vi "GraphChartFactory.vi"(8 "error in":errorcluster, 11 "Gen Refnum":refnum<vi>) -> (0 "error out":errorcluster, 3 "GraphChart out":refnum<class "GraphChart.lvclass">)   [LabVIEW 2014, in "GraphChart.lvclass"]
uses:
  GraphChart.lvclass
  WaveformChart/WaveformChart.lvclass
  WaveformGraph/WaveformGraph.lvclass
  XYGraph/XYGraph.lvclass
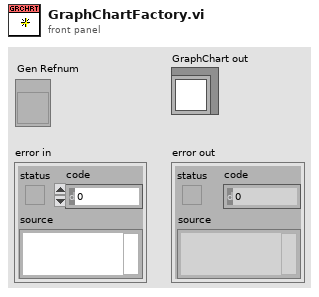
[diagram p1: front panel]
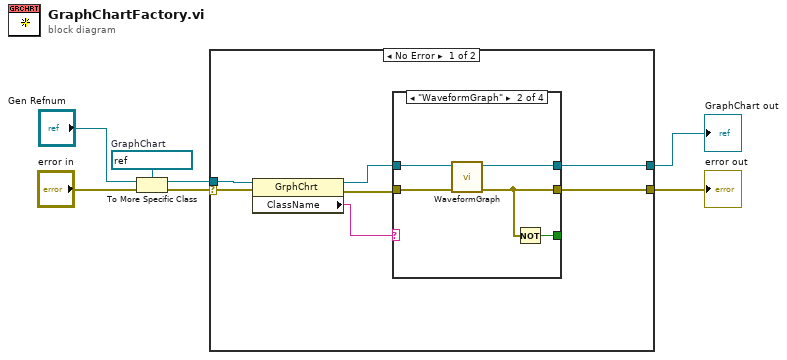
[diagram p0: block diagram]
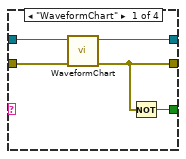
[diagram p2: hidden frame]
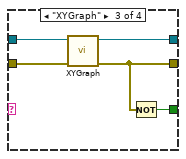
[diagram p3: hidden frame]
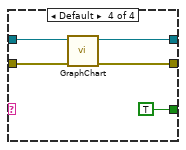
[diagram p4: hidden frame]
diagram:
  w5 = refnum<vi> refnum  # GraphChart
  n1 = To More Specific Class(target class=w5, reference="Gen Refnum", error in="error in") -> (specific class reference=w3:refnum<vi>, error out=w4:errorcluster)
  n2 = case shown="No Error" w4 {
    selector: w4 -> [w12 w35]
    tunnel: [w14 _] -> w1
    tunnel: [w13 w35] -> w2
    tunnel: w3 -> [w11 _]
    frame No Error {
      n3 = property class="GrphChrt"(reference=w11, error in=w12) -> (reference out=w8:refnum<vi>, error out=w9:errorcluster, "ClassName"=w10:string)
      n4 = case shown="\"WaveformGraph\"" w10 {
        tunnel: w9 -> [w19 w24 w29 w32]
        tunnel: [w16 w21 w26 w30] -> w13
        tunnel: [w18 w23 w28 w31] -> w14
        tunnel: [w17 w22 w27 TRUE] -> _
        tunnel: w8 -> [w15 w20 w25 w33]
        frame "WaveformChart" {
          n5 = call "WaveformChart.vi"("error in"=w19, "Gen Refnum"=w15) -> ("error out"=w16:errorcluster, "WFChart out"=w18:refnum<class "WaveformChart.lvclass">)  [unwired: 8 in]
          n6 = Not(x=w16) -> (.not. x?=w17:bool)
        }
        frame "WaveformGraph" {
          n7 = call "WaveformGraph.vi"("error in"=w24, "Gen Refnum"=w20) -> ("error out"=w21:errorcluster, "WFGraph out"=w23:refnum<class "WaveformGraph.lvclass">)  [unwired: 8 in]
          n8 = Not(x=w21) -> (.not. x?=w22:bool)
        }
        frame "XYGraph" {
          n9 = call "XYGraph.vi"("error in"=w29, "Gen Refnum"=w25) -> ("error out"=w26:errorcluster, "XYGraph out"=w28:refnum<class "XYGraph.lvclass">)  [unwired: 8 in]
          n10 = Not(x=w26) -> (.not. x?=w27:bool)
        }
        frame Default {
          n11 = call "GraphChart.vi"("error in"=w32, "Gen Refnum"=w33) -> ("error out"=w30:errorcluster, "GraphChart out"=w31:refnum<class "GraphChart.lvclass">)  [unwired: 8 in]
        }
      }
    }
    frame Error {
    }
  }
  "error out" <- w2
  "GraphChart out" <- w1
